vi "test_DMA Channels Input.vi"(8 "error in (no error)":errorcluster, 11 "TestCase in":refnum<class "DMA Channel Testing.lvclass">) -> (0 "error out":errorcluster, 3 "TestCase out":refnum<class "DMA Channel Testing.lvclass">)   [LabVIEW 2019, in "DMA Channel Testing.lvclass"]
uses:
  DMA Channel Testing.lvclass
  Addon/Addon Shared/Types/DMA Settings.ctl
  Addon/Addon Shared/Types/Delacing Scheme.ctl
  Addon/Addon Shared/Types/DMA Acquisition Mode.ctl
  DMA Channel Testing.lvclass/DMA Channel Testing.ctl
  Addon/Addon Shared/SubVIs/Constants.vi
  <vilib>/NI/NI VeriStand Advanced SysDef API/_SubVIs/SysDef.Search.GUID.vi
  <vilib>/NI/NI VeriStand Advanced SysDef API/_SubVIs/SysDef.Search.GUIDs.vi
  <vilib>/addons/_JKI Toolkits/VI Tester/TestCase.llb/TestCase.lvclass
  Addon/Addon System Explorer/FPGA Addon System Explorer.lvlib
  Addon/Addon Shared/FPGA Addon Shared.lvlib
  <vilib>/NI/NI VeriStand Advanced SysDef API/SysDef API/Advanced System Definition.lvlib
  C:/Program Files (x86)/National Instruments/LabVIEW 2019/vi.lib/addons/_JKI Toolkits/VI Tester/TestCase.llb/TestCase.lvclass
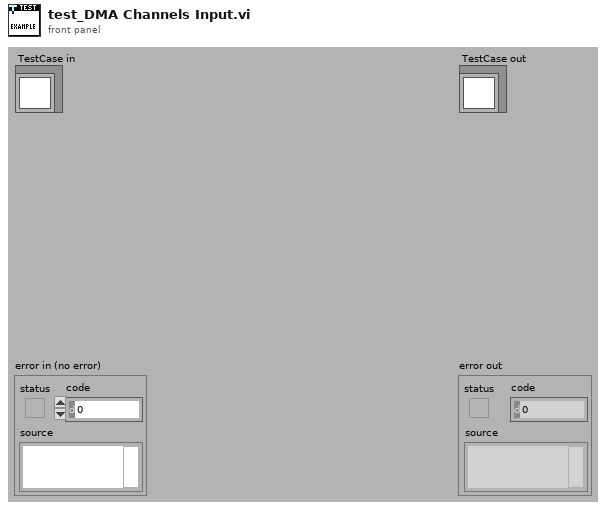
[diagram p1: front panel]
types:
  T1 = typedef "FPGA Addon Shared.lvlib/DMA Settings.ctl" = cluster{"Number of Channels":u8, "Delacing Scheme":T2, "Update Rate":u32, "dt":dbl, "Mode":T3, "Number of Samples":u32, "DMA Host Buffer":u32}
  T2 = typedef "FPGA Addon Shared.lvlib/Delacing Scheme.ctl" = enum8{"Interleaved", "Bitpacked"}
  T3 = typedef "FPGA Addon Shared.lvlib/DMA Acquisition Mode.ctl" = enum8{"Continuous", "Triggered Finite"}
  T4 = typedef "Advanced System Definition.lvlib/TreeItem.Info.ctl" = cluster{"Name":string, "Description":string, "GUID":string, "Is Channel":bool, "Channel":T5, "Is Waveform":bool, "Waveform":T7}
  T5 = typedef "Custom Device API.lvlib/Custom Device Channel.ctl" = cluster{"Type":T6, "Units":string, "Default Value":dbl, "Faultable":bool, "Scalable":bool}
  T6 = typedef "Custom Device API.lvlib/Custom Device Channel Type.ctl" = enum16{"Input", "Output"}
  T7 = typedef "Custom Device API.lvlib/Custom Device Waveform.ctl" = cluster{"Data Type":T8, "Units":string}
  T8 = typedef "Custom Device API.lvlib/Custom Device Waveform DataType.ctl" = enum16{"Double", "Complex Double"}
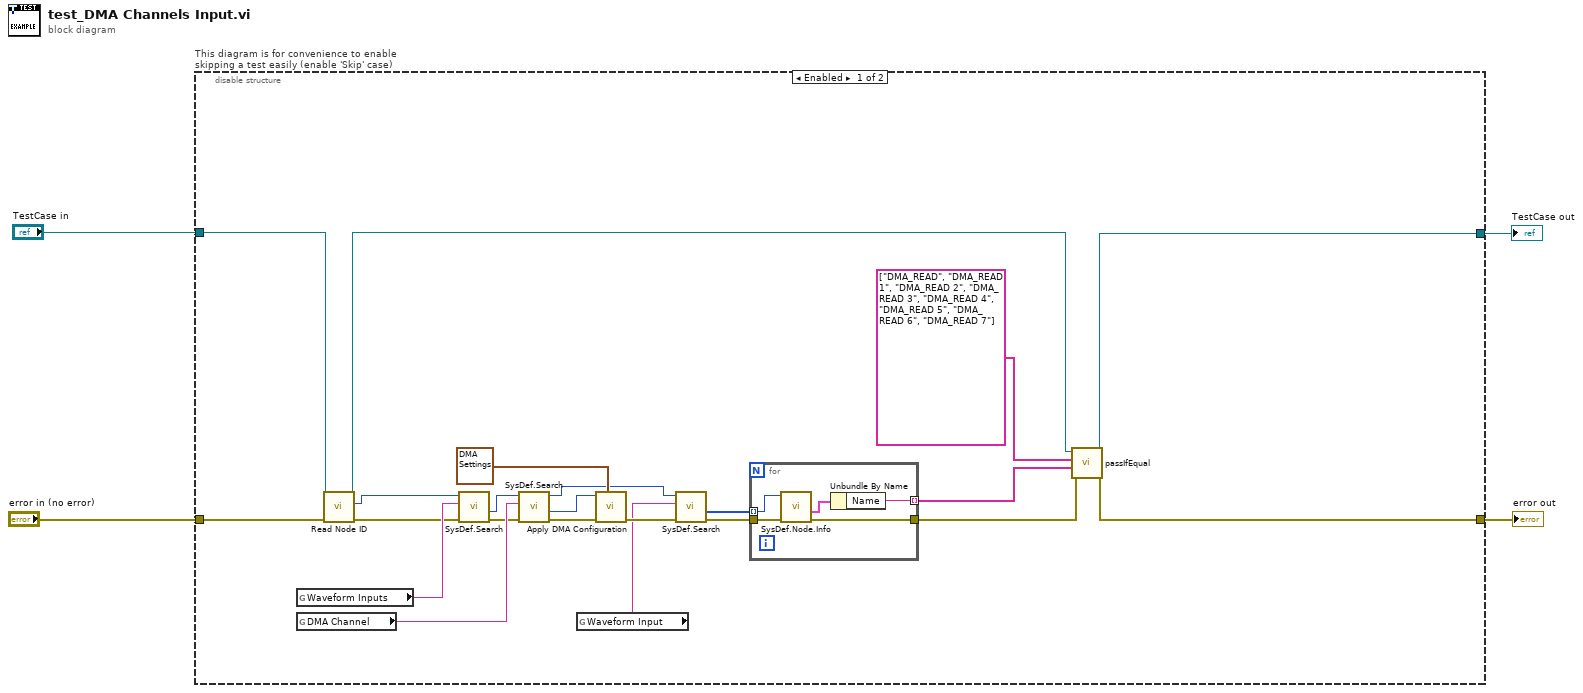
[diagram p0: block diagram]
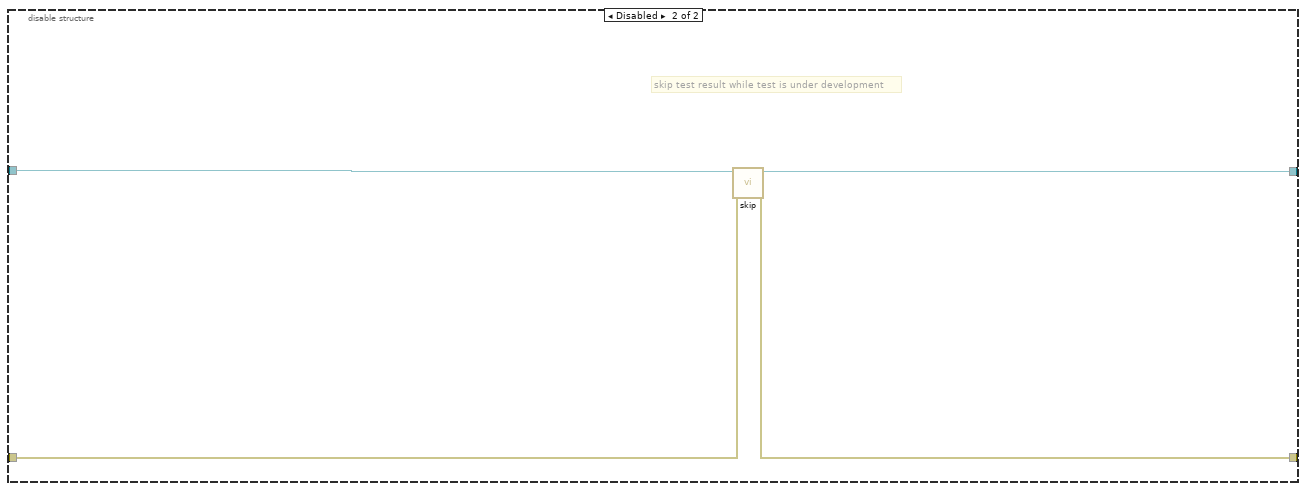
[diagram p2: hidden frame]
diagram:
  n1 = disable-structure "This diagram is for convenience to enable skipping a test easily (enable 'Skip' case)" shown="Enabled" {
    disable-tunnel: "TestCase in" -> [w5 w35]
    disable-tunnel: [w26 w33] -> w1
    disable-tunnel: [w25 w34] -> w3
    disable-tunnel: "error in (no error)" -> [w9 w32]
    frame Enabled {
      n2 = global read "Constants.vi" "Waveform Inputs"() -> (w22:string)
      n3 = global read "Constants.vi" "DMA Channel"() -> (w21:string)
      n4 = call "Read Node ID.vi"("error in (no error)"=w9, "DMA Channel Testing in"=w5) -> ("error out"=w8:errorcluster, "Node ID"=w7:u64, "DMA Channel Testing out"=w6:refnum<class "DMA Channel Testing.lvclass">)  [unwired: 7 in]
      n5 = call-poly <vilib>:"SysDef.Search.vi"("error in (no error)"=w8, "GUID"=w22, "nodeID"=w7) -> ("error out"=w19:errorcluster, "Value out"=w20:u64)  [unwired: 5 in, 2 out]
      n6 = call-poly <vilib>:"SysDef.Search.vi"("error in (no error)"=w19, "GUID"=w21, "nodeID"=w20) -> ("error out"=w23:errorcluster, "Value out"=w18:u64, "nodeID out"=w15:u64)  [unwired: 5 in, 1 out]
      n7 = global read "Constants.vi" "Waveform Input"() -> (w16:string)
      n8 = call "Apply DMA Configuration.vi"("DMA Settings"=T1 {"Number of Channels"=8, "Delacing Scheme"=enum."Interleaved", "Update Rate"=0, "dt"=0.0, "Mode"=enum."Continuous", "Number of Samples"=0, "DMA Host Buffer"=0}, "error in (no error)"=w23, "Item Ref in"=w18) -> ("error out"=w17:errorcluster)  [unwired: 8 in]
      n9 = call-poly <vilib>:"SysDef.Search.vi"("error in (no error)"=w17, "GUID"=w16, "nodeID"=w15) -> ("error out"=w13:errorcluster, "Values Out"=w14:u64[])  [unwired: 5 in, 2 out]
      n10 = for {
        tunnel: w14 -> [w31] mode=indexing
        tunnel: w13 -> [w30]
        tunnel: [w29] -> w12
        tunnel: [w27] -> w11 mode=indexing
        n11 = call <vilib>:"SysDef.Node.Info.vi"("error in (no error)"=w30, "nodeID"=w31) -> ("error out"=w29:errorcluster, "Item Info"=w28:T4)  [unwired: 6 in, 2 out]
        n12 = Unbundle By Name(w28) -> ("Name"=w27:string)
      }
      n13 = call-dynamic "passIfEqual.vi"("error in (no error)"=w12, "y"=w11, "x"=string[] ["DMA_READ", "DMA_READ 1", "DMA_READ 2", "DMA_READ 3", "DMA_READ 4", "DMA_READ 5", "DMA_READ 6", "DMA_READ 7"] ("Array"), "TestCase in"=w6) -> ("error out"=w25:errorcluster, "TestCase out"=w26:refnum<class "DMA Channel Testing.lvclass">)  [unwired: 6 in]
    }
    frame Disabled {
      # "skip test result while test is under development"
      n14 = call <vilib>:"skip.vi"("error in (no error)"=w32, "TestCase in"=w35) -> ("error out"=w34:errorcluster, "TestCase out"=w33:refnum<class "DMA Channel Testing.lvclass">)  [unwired: 8 in]
    }
  }
  "error out" <- w3
  "TestCase out" <- w1
